vi "Read.vi"(8 "error in (no error)":errorcluster, 11 "ConvertTo in":refnum<class "ConvertTo_U16.lvclass">) -> (0 "error out":errorcluster, 2 "Value":u16, 3 "ConvertTo out":refnum<class "ConvertTo_U16.lvclass">)   [LabVIEW 2021, in "ConvertTo_U16.lvclass"]
uses:
  ConvertTo_U16.lvclass
  ConvertTo_U16.lvclass/ConvertTo_U16.ctl
  Properties/Read Value.vi
  Properties/Write Value.vi
  Abs_Types/Numeric/Abs_Numeric.lvclass
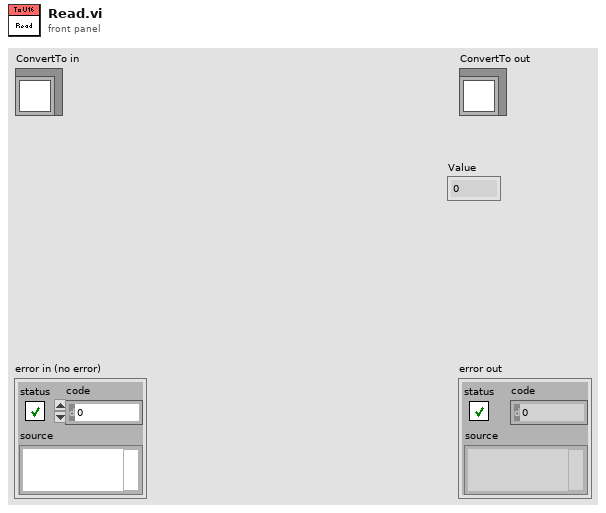
[diagram p1: front panel]
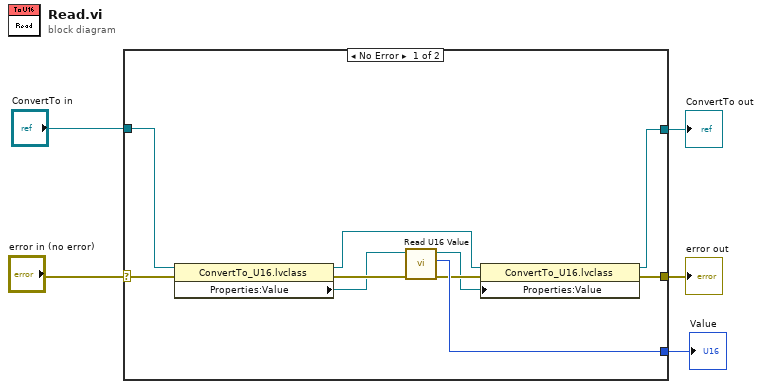
[diagram p0: block diagram]
diagram:
  n1 = case shown="No Error" "error in (no error)" {
    selector: "error in (no error)" -> [w15 w16]
    tunnel: "ConvertTo in" -> [w14 w17]
    tunnel: [w11 _] -> w3
    tunnel: [w7 w16] -> w2
    tunnel: [w6 w17] -> w1
    frame No Error {
      n2 = property class="ConvertTo_U16.lvclass"(reference=w14, error in=w15) -> (reference out=w10:refnum<class "ConvertTo_U16.lvclass">, error out=w13:errorcluster, "Properties:Value"=w12:refnum<class "Abs_Numeric.lvclass">)
      n3 = call-dynamic "Read U16 Value.vi"("error in (no error)"=w13, "Numeric in"=w12) -> ("error out"=w9:errorcluster, "U16"=w11:u16, "Numeric out"=w8:refnum<class "Abs_Numeric.lvclass">)  [unwired: 7 in]
      n4 = property class="ConvertTo_U16.lvclass"(reference=w10, error in=w9, "Properties:Value"=w8) -> (reference out=w6:refnum<class "ConvertTo_U16.lvclass">, error out=w7:errorcluster)
    }
    frame Error {
    }
  }
  "error out" <- w2
  "ConvertTo out" <- w1
  "Value" <- w3
